vi "Pre-Uninstall Action.vi"   [LabVIEW 2013]
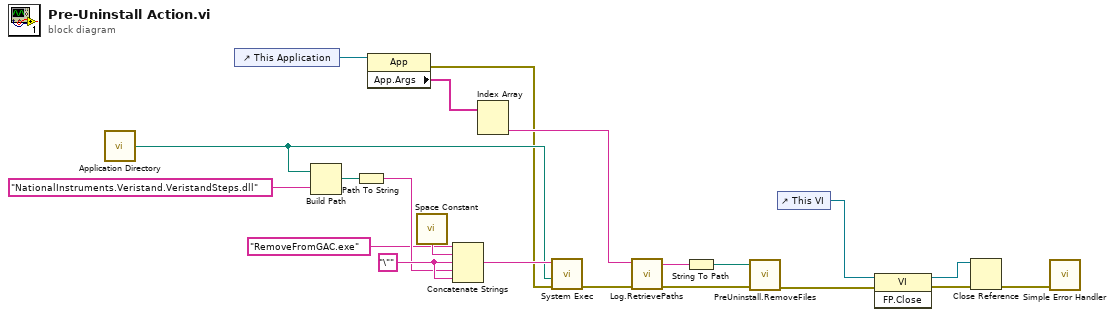
[diagram p0: block diagram]
diagram:
  w21 = "\"" ("string")
  n1 = call <vilib>:"Application Directory.vi"() -> ("Application Directory"=w14:path)
  n2 = control-ref of="This Application"() -> (w4:refnum<vi>)
  n3 = Build Path(base path=w14, name or relative path="NationalInstruments.Veristand.VeristandSteps.dll" ("command line")) -> (appended path=w19:path)
  n4 = Path To String(path=w19) -> (string=w17:string)
  n5 = property class="App"(reference=w4) -> (error out=w1:errorcluster, "App.Args"=w3:string[])  [unwired: 1 in, 1 out]
  n6 = call <vilib>:"Space Constant.vi"() -> ("String"=w20:string)
  n7 = Concatenate Strings("RemoveFromGAC.exe" ("string"), w20, w21, w17, w21) -> (w15:string)
  n8 = Index Array(array=w3) -> (element #2=w2:string)  [unwired: 2 in, 1 out]
  n9 = call <vilib>:"System Exec.vi"("error in (no error)"=w1, "working directory"=w14, "command line"=w15) -> ("error out"=w9:errorcluster)  [unwired: 5 in, 3 out]
  n10 = call "Log.RetrievePaths.vi"("error in (no error)"=w9, "VeriStand Version (2013 SP1)"=w2) -> ("error out"=w8:errorcluster, "TestStand Install Directory"=w6:string)  [unwired: 8 in]
  n11 = String To Path(string=w6) -> (path=w5:path)
  n12 = call "PreUninstall.RemoveFiles.vi"("error in (no error)"=w8, "TestStand Components\\TypePalettes Directory"=w5) -> ("error out"=w7:errorcluster)  [unwired: 9 in]
  n13 = control-ref of="This VI"() -> (w13:refnum<vi>)
  n14 = invoke class="VI" method="FP.Close"(reference=w13, error in=w7) -> (reference out=w11:refnum<vi>, error out=w12:errorcluster)  [unwired: 1 in, 1 out]
  n15 = Close Reference(reference=w11, error in (no error)=w12) -> (error out=w10:errorcluster)
  n16 = call <vilib>:"Simple Error Handler.vi"("error in (no error)"=w10) -> ()  [unwired: 4 in, 5 out]
